vi "TRDU_DBC.vi"(10 "Datain":T1, 11 "TRDU CLUSTER IN in":T2) -> (2 "x = y?":bool, 3 "TRDU CLUSTER IN out":T2)   [LabVIEW 2020]
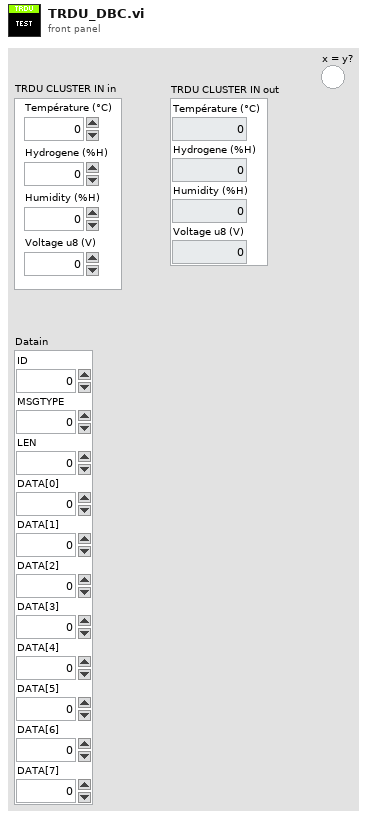
[diagram p1: front panel]
types:
  T1 = cluster{"ID":u32, "MSGTYPE":u8, "LEN":u8, "DATA[0]":u8, "DATA[1]":u8, "DATA[2]":u8, "DATA[3]":u8, "DATA[4]":u8, "DATA[5]":u8, "DATA[6]":u8, "DATA[7]":u8}
  T2 = cluster{"Température (°C)":dbl, "Hydrogene (%H)":dbl, "Humidity (%H)":dbl, "Voltage u8 (V)":dbl}
  T3 = cluster{"DATA[0]":u8, "DATA[1]":u8, "DATA[2]":u8, "DATA[3]":u8, "DATA[4]":u8, "DATA[5]":u8, "DATA[6]":u8, "DATA[7]":u8}
  T4 = cluster{"[0]":u8, "[1]":u8, "[2]":u8, "[3]":u8, "[4]":u8, "[5]":u8, "[6]":u8, "[7]":u8}
  T5 = cluster{"Boolean array[0]":bool, "Boolean array[1]":bool, "Boolean array[2]":bool, "Boolean array[3]":bool, "Boolean array[4]":bool, "Boolean array[5]":bool, "Boolean array[6]":bool, "Boolean array[7]":bool}
  T6 = cluster{"Boolean array[0]":bool, "Boolean array[1]":bool, "Boolean array[2]":bool, "Boolean array[3]":bool, "Boolean array[4]":bool, "Boolean array[5]":bool, "Boolean array[6]":bool, "Boolean array[7]":bool, "Boolean array[0]":bool, "Boolean array[1]":bool, "Boolean array[2]":bool, "Boolean array[3]":bool, "Boolean array[4]":bool, "Boolean array[5]":bool, "Boolean array[6]":bool, "Boolean array[7]":bool}
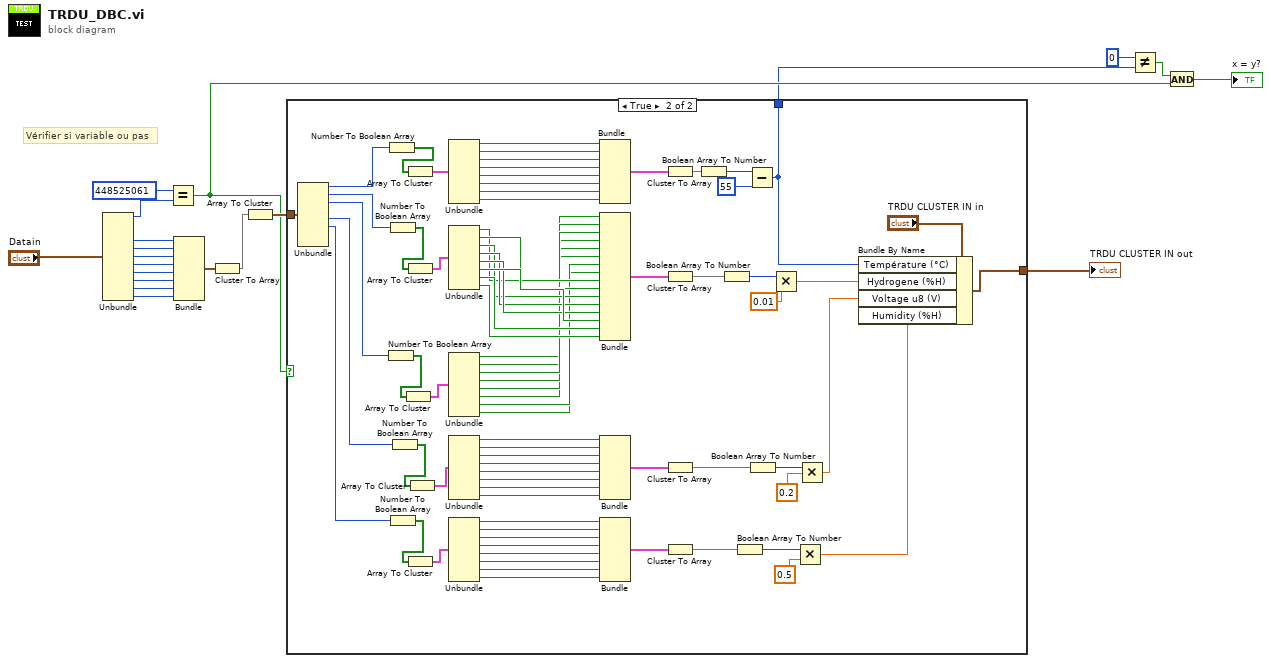
[diagram p0: block diagram]
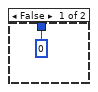
[diagram p2: hidden frame]
diagram:
  # "Vérifier si variable ou pas"
  n1 = Unbundle("Datain") -> ("ID"=w7:u32, "DATA[0]"=w9:u8, "DATA[1]"=w10:u8, "DATA[2]"=w11:u8, "DATA[3]"=w13:u8, "DATA[4]"=w12:u8, "DATA[5]"=w14:u8, "DATA[6]"=w15:u8, "DATA[7]"=w16:u8)  [unwired: 2 out]
  n2 = Equal?(x=u32 448525061, y=w7) -> (x = y?=w5:bool)
  n3 = Bundle("DATA[0]"=w9, "DATA[1]"=w10, "DATA[2]"=w11, "DATA[3]"=w13, "DATA[4]"=w12, "DATA[5]"=w14, "DATA[6]"=w15, "DATA[7]"=w16) -> (w18:T3)  [unwired: 1 in]
  n4 = Cluster To Array(cluster=w18) -> (array=w19:u8[])
  n5 = Array To Cluster(array=w19) -> (cluster=w17:T4)
  n6 = case shown="True" w5 {
    tunnel: [_ w23] -> w20
    tunnel: w17 -> [_ w28]
    tunnel: [u32 0 w22] -> w2
    frame False {
    }
    frame True {
      n7 = Unbundle(w28) -> ("[0]"=w31:u8, "[1]"=w32:u8, "[2]"=w24:u8, "[4]"=w69:u8, "[5]"=w70:u8)  [unwired: 3 out]
      n8 = Number To Boolean Array(number=w24) -> (Boolean array=w25:bool[])
      n9 = Number To Boolean Array(number=w31) -> (Boolean array=w30:bool[])
      n10 = Number To Boolean Array(number=w32) -> (Boolean array=w27:bool[])
      n11 = Number To Boolean Array(number=w70) -> (Boolean array=w68:bool[])
      n12 = Number To Boolean Array(number=w69) -> (Boolean array=w67:bool[])
      n13 = Array To Cluster(array=w25) -> (cluster=w54:T5)
      n14 = Array To Cluster(array=w30) -> (cluster=w29:T5)
      n15 = Array To Cluster(array=w27) -> (cluster=w45:T5)
      n16 = Array To Cluster(array=w68) -> (cluster=w88:T5)
      n17 = Array To Cluster(array=w67) -> (cluster=w87:T5)
      n18 = Unbundle(w29) -> ("Boolean array[0]"=w33:bool, "Boolean array[1]"=w34:bool, "Boolean array[2]"=w40:bool, "Boolean array[3]"=w39:bool, "Boolean array[4]"=w38:bool, "Boolean array[5]"=w37:bool, "Boolean array[6]"=w36:bool, "Boolean array[7]"=w35:bool)
      n19 = Unbundle(w45) -> ("Boolean array[0]"=w55:bool, "Boolean array[1]"=w56:bool, "Boolean array[2]"=w57:bool, "Boolean array[3]"=w58:bool, "Boolean array[4]"=w59:bool, "Boolean array[5]"=w60:bool, "Boolean array[6]"=w61:bool, "Boolean array[7]"=w99:bool)
      n20 = Unbundle(w54) -> ("Boolean array[0]"=w46:bool, "Boolean array[1]"=w47:bool, "Boolean array[2]"=w53:bool, "Boolean array[3]"=w52:bool, "Boolean array[4]"=w51:bool, "Boolean array[5]"=w50:bool, "Boolean array[6]"=w49:bool, "Boolean array[7]"=w48:bool)
      n21 = Unbundle(w87) -> ("Boolean array[0]"=w78:bool, "Boolean array[1]"=w77:bool, "Boolean array[2]"=w71:bool, "Boolean array[3]"=w72:bool, "Boolean array[4]"=w73:bool, "Boolean array[5]"=w74:bool, "Boolean array[6]"=w75:bool, "Boolean array[7]"=w76:bool)
      n22 = Unbundle(w88) -> ("Boolean array[0]"=w79:bool, "Boolean array[1]"=w80:bool, "Boolean array[2]"=w86:bool, "Boolean array[3]"=w85:bool, "Boolean array[4]"=w84:bool, "Boolean array[5]"=w83:bool, "Boolean array[6]"=w82:bool, "Boolean array[7]"=w81:bool)
      n23 = Bundle("Boolean array[0]"=w33, "Boolean array[1]"=w34, "Boolean array[2]"=w40, "Boolean array[3]"=w39, "Boolean array[4]"=w38, "Boolean array[5]"=w37, "Boolean array[6]"=w36, "Boolean array[7]"=w35) -> (w41:T5)  [unwired: 1 in]
      n24 = Bundle("Boolean array[0]"=w46, "Boolean array[1]"=w47, "Boolean array[2]"=w53, "Boolean array[3]"=w52, "Boolean array[4]"=w51, "Boolean array[5]"=w50, "Boolean array[6]"=w49, "Boolean array[7]"=w48, "Boolean array[0]"=w55, "Boolean array[1]"=w56, "Boolean array[2]"=w57, "Boolean array[3]"=w58, "Boolean array[4]"=w59, "Boolean array[5]"=w60, "Boolean array[6]"=w61, "Boolean array[7]"=w99) -> (w62:T6)  [unwired: 1 in]
      n25 = Bundle("Boolean array[0]"=w78, "Boolean array[1]"=w77, "Boolean array[2]"=w71, "Boolean array[3]"=w72, "Boolean array[4]"=w73, "Boolean array[5]"=w74, "Boolean array[6]"=w75, "Boolean array[7]"=w76) -> (w96:T5)  [unwired: 1 in]
      n26 = Bundle("Boolean array[0]"=w79, "Boolean array[1]"=w80, "Boolean array[2]"=w86, "Boolean array[3]"=w85, "Boolean array[4]"=w84, "Boolean array[5]"=w83, "Boolean array[6]"=w82, "Boolean array[7]"=w81) -> (w92:T5)  [unwired: 1 in]
      n27 = Cluster To Array(cluster=w41) -> (array=w26:bool[])
      n28 = Cluster To Array(cluster=w62) -> (array=w63:bool[])
      n29 = Cluster To Array(cluster=w96) -> (array=w93:bool[])
      n30 = Cluster To Array(cluster=w92) -> (array=w91:bool[])
      n31 = Boolean Array To Number(Boolean array=w26) -> (number=w42:u32)
      n32 = Boolean Array To Number(Boolean array=w63) -> (number=w64:u32)
      n33 = Boolean Array To Number(Boolean array=w91) -> (number=w90:u32)
      n34 = Subtract(x=w42, y=u32 55) -> (x-y=w22:u32)
      n35 = Boolean Array To Number(Boolean array=w93) -> (number=w94:u32)
      n36 = Multiply(x=w64, y=0.01) -> (x*y=w66:dbl)
      n37 = Multiply(x=w90, y=0.5) -> (x*y=w98:dbl)
      n38 = Multiply(x=w94, y=0.2) -> (x*y=w97:dbl)
      n39 = Bundle By Name(cluster="TRDU CLUSTER IN in", "Température (°C)"=w22, "Hydrogene (%H)"=w66, "Voltage u8 (V)"=w97, "Humidity (%H)"=w98) -> (w23:T2)
    }
  }
  "TRDU CLUSTER IN out" <- w20
  n40 = Not Equal?(x=u32 0, y=w2) -> (x != y?=w3:bool)
  n41 = And(x=w3, y=w5) -> (x .and. y?=→"x = y?":bool)
